vi "Check and send command to corresponding device.vi"(8 "error in (no error)":errorcluster, 9 "Execute cmd (F)":bool, 10 "Cmd string":string="power -10 0") -> (0 "error out":errorcluster, 3 "Response":string)   [LabVIEW 2019]
doc: "Nicolas Weiss - EPFL - IPHYS 2019\n----\nThis VI :\n- parses a user command\n- checks syntax and arguments validity\n- sends it to the corresponding device"
uses:
  Controls/Log destination selector.ctl
  Controls/Lakeshore device selector.ctl
  _Global variables 1.vi
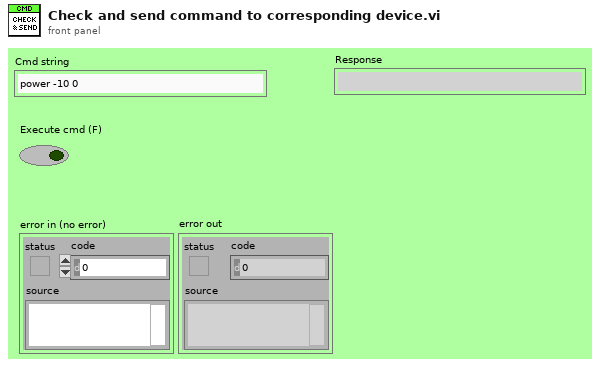
[diagram p1: front panel]
types:
  T1 = typedef "Log destination selector.ctl" = enum16{"UI", "File", "UI+file"}
  T2 = typedef "Lakeshore device selector.ctl" = enum16{"A", "B"}
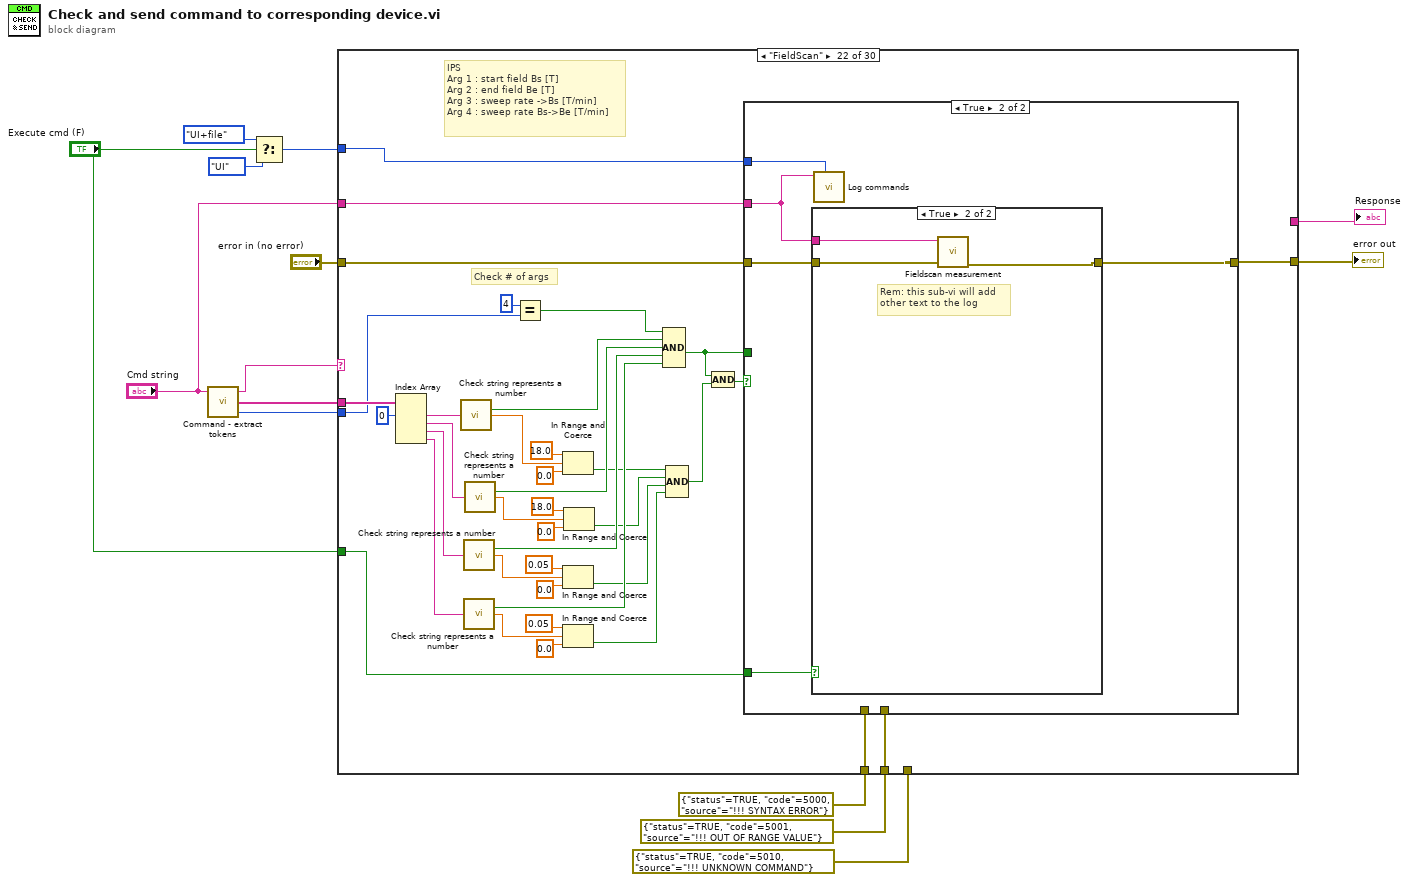
[diagram p0: block diagram]
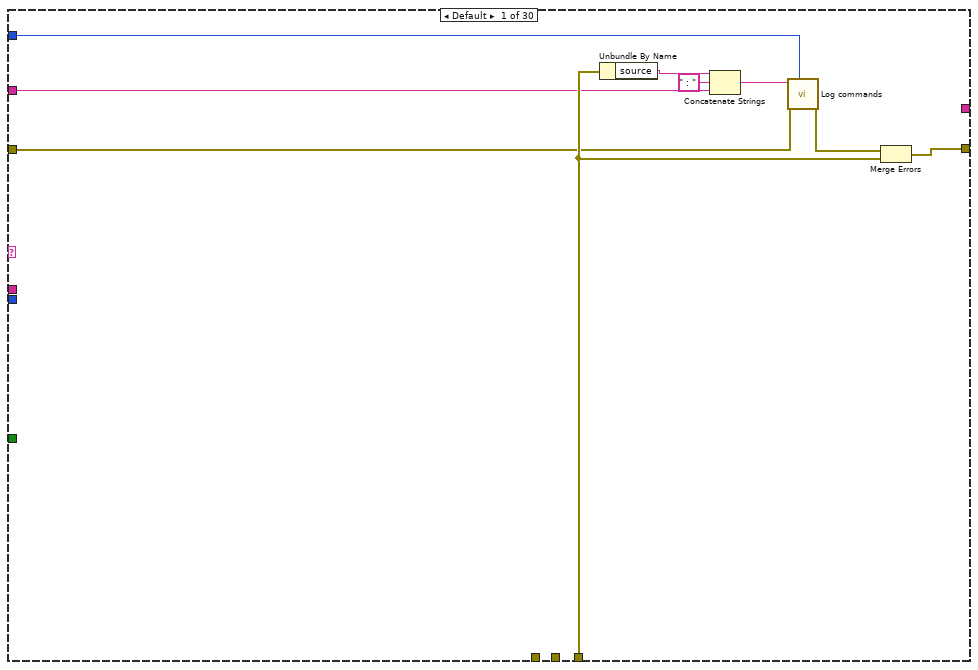
[diagram p2: hidden frame]
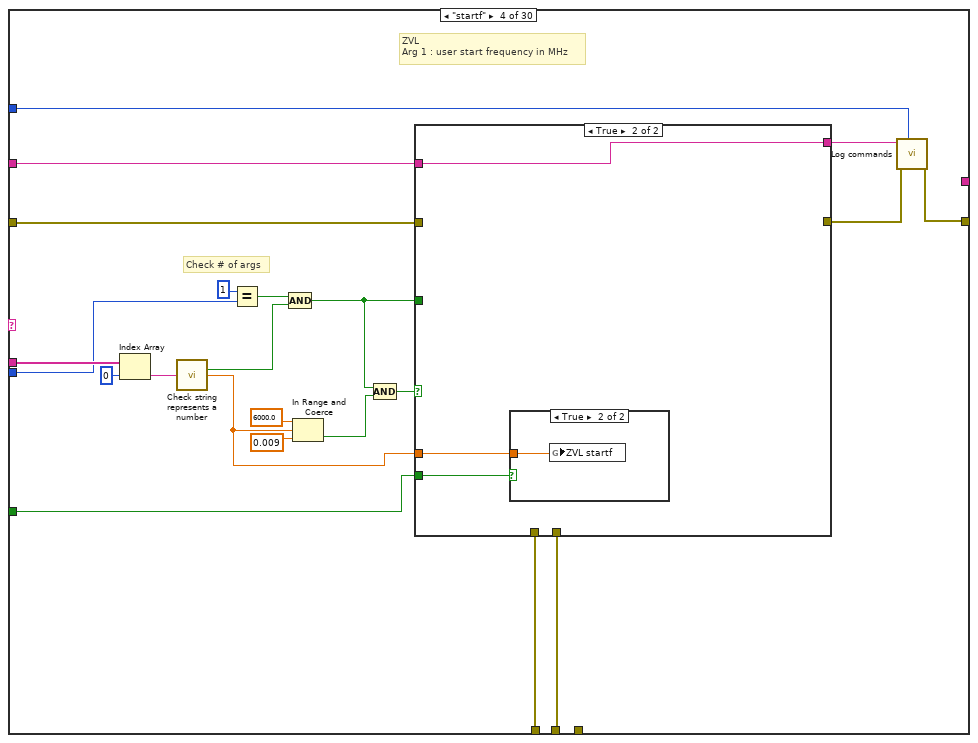
[diagram p5: hidden frame]
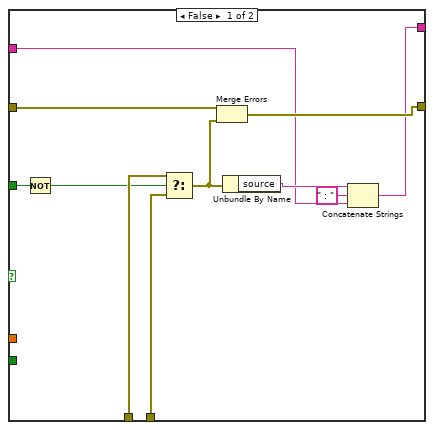
[diagram p6: hidden frame]
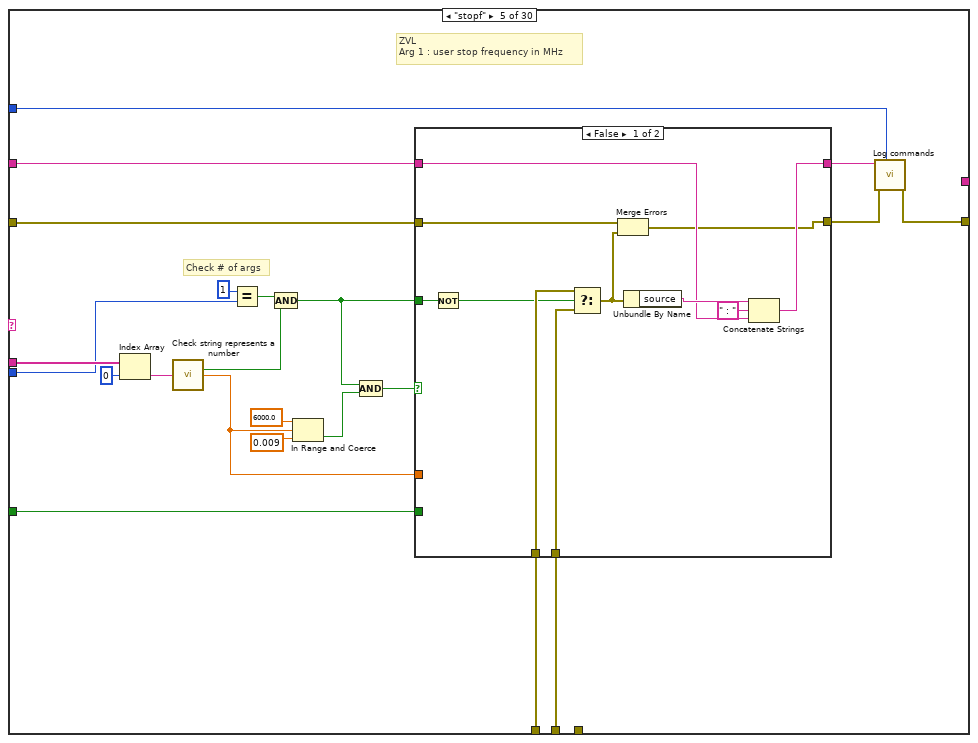
[diagram p8: hidden frame]
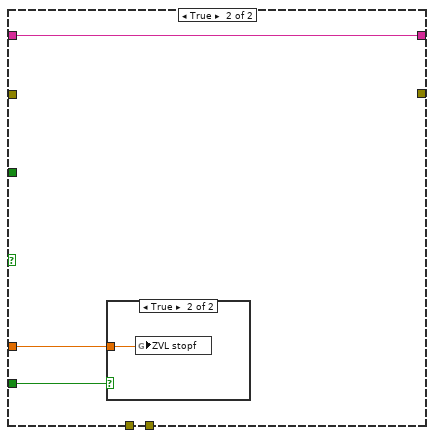
[diagram p9: hidden frame]
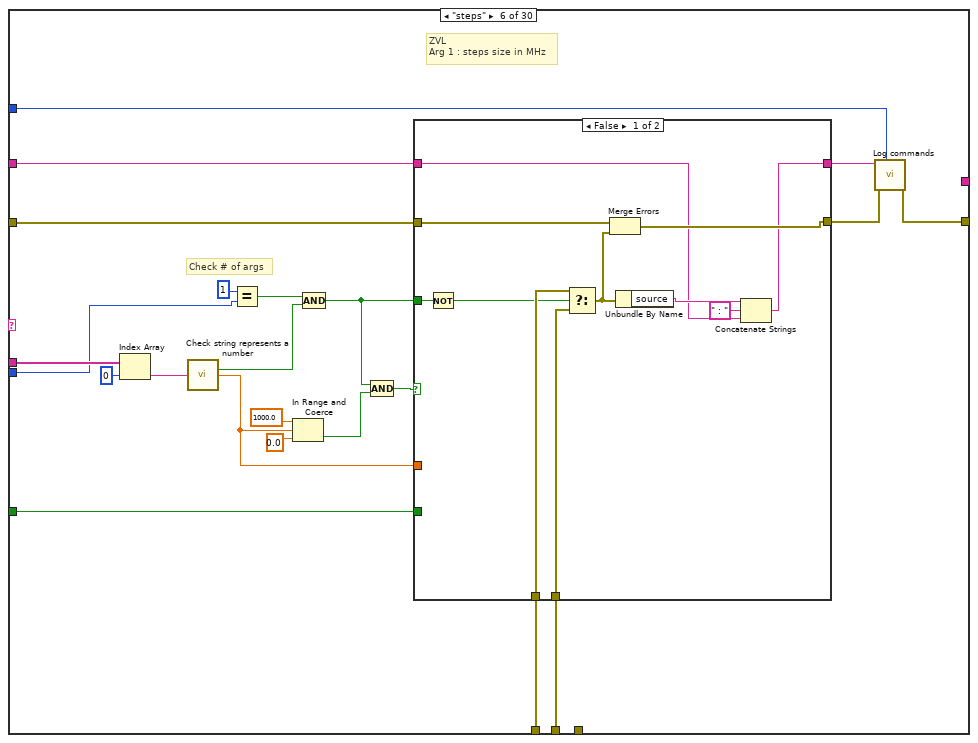
[diagram p11: hidden frame]
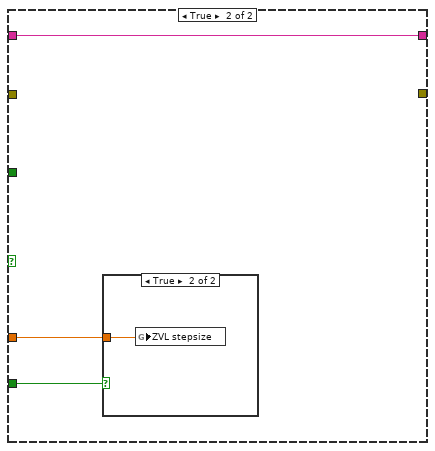
[diagram p12: hidden frame]
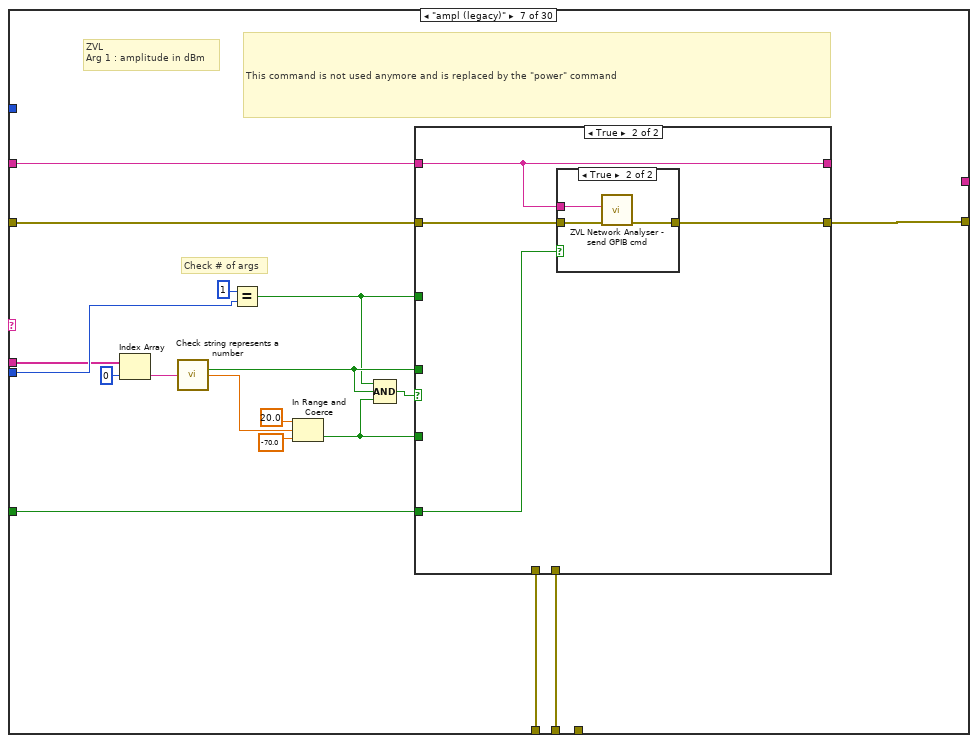
[diagram p14: hidden frame]
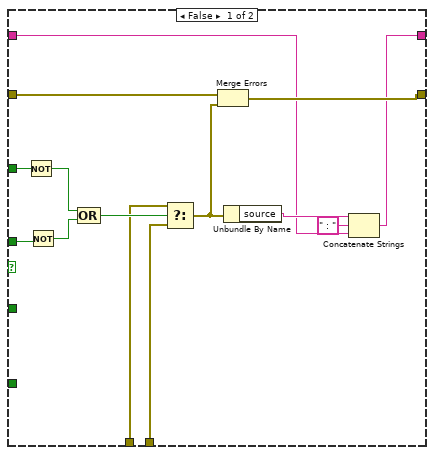
[diagram p15: hidden frame]
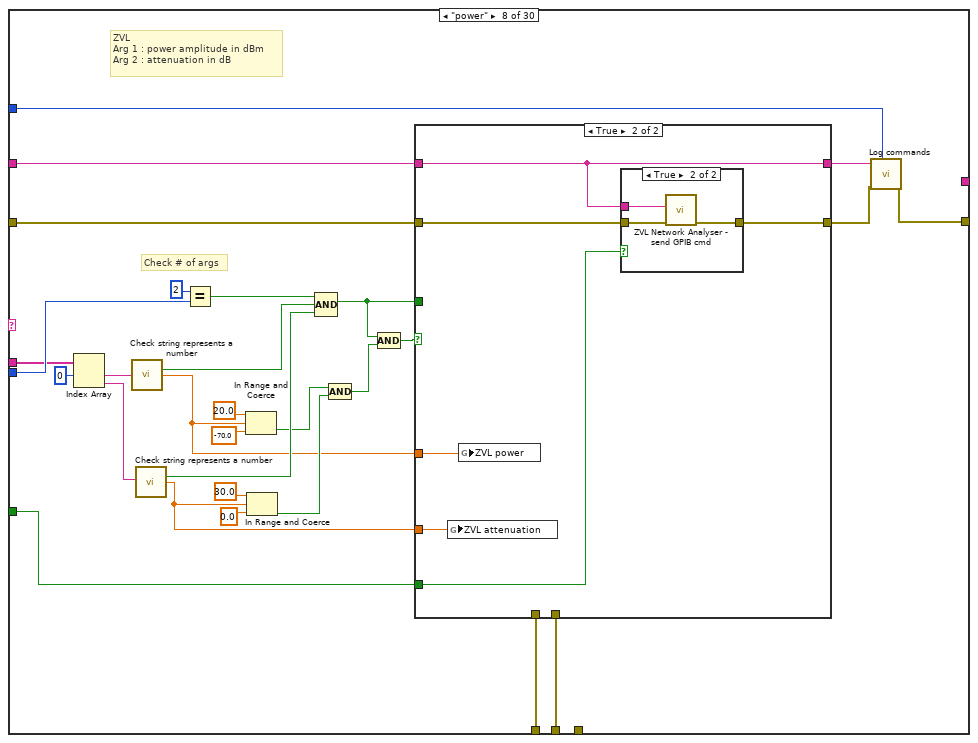
[diagram p17: hidden frame]
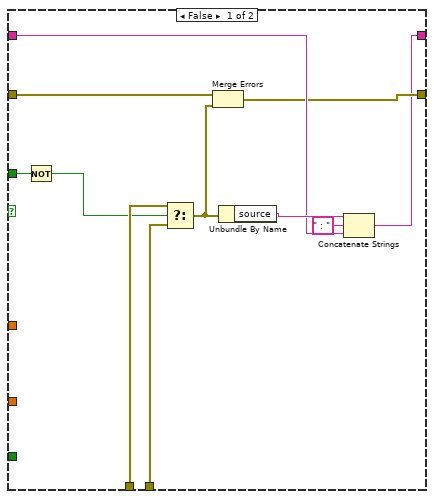
[diagram p18: hidden frame]
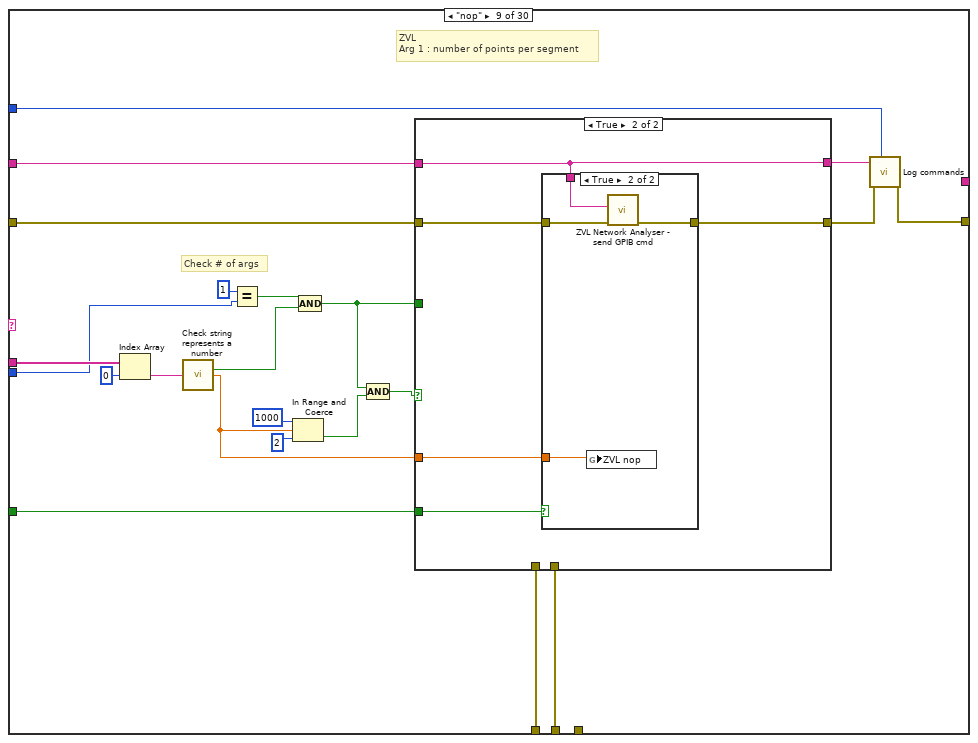
[diagram p20: hidden frame]
diagram:
  n1 = call "Command - extract tokens.vi"("Cmd string"="Cmd string") -> ("N arg"=w8:u8, "Arguments"=w11:string[], "Command"=w9:string)  [unwired: 2 in]
  n2 = Select(t=Log_destination_selector."UI+file" ("Log destination"), s="Execute cmd (F)", f=Log_destination_selector."UI" ("Log destination")) -> (s? t:f=w1:T1)
  n3 = case shown="\"FieldScan\"" w9 {
    tunnel: w11 -> [_ _ _ w46 w83 w120 w151 w199 w247 _ _ _ w308 w348 w383 _ _ _ _ _ _ w596 _ w647 w687 _ _ _ _ _]
    tunnel: w8 -> [_ _ _ w44 w82 w119 w154 w204 w246 _ _ _ w307 w347 w382 w411 w438 w467 w496 w524 w550 w585 _ w646 w686 _ _ _ _ _]
    tunnel: "error in (no error)" -> [w16 w24 w25 w40 w78 w115 w153 w200 w242 w272 w281 w287 w303 w343 w380 w409 w436 w465 w494 w522 w548 w598 w626 w642 w682 w710 w720 w727 w728 w729]
    tunnel: [w23 w24 w25 w30 w68 w105 w152 w177 w232 w271 w280 w287 w293 w333 w372 w401 w428 w457 w486 w514 w540 w597 w626 w632 w672 w709 w719 w727 w728 w729] -> w13
    tunnel: [_ _ _ _ _ _ _ _ _ w270 w279 _ _ _ _ _ w426 w455 w484 _ _ _ _ _ _ w708 w718 _ _ _] -> w12
    tunnel: "Cmd string" -> [w19 _ _ w39 w77 w114 w150 w198 w241 _ _ _ w302 w342 w379 w408 w435 w464 w493 w521 w547 w595 _ w641 w681 _ _ _ _ _]
    tunnel: "Execute cmd (F)" -> [_ _ _ w38 w76 w113 w149 w197 w240 w269 w278 _ w301 w341 w378 w407 w434 w463 w492 w520 w546 w594 _ w640 w680 w707 w717 _ _ _]
    tunnel: errorcluster {"status"=TRUE, "code"=5001, "source"="!!! OUT OF RANGE VALUE"} ("error out") -> [_ _ _ w34 w72 w110 w147 w194 w236 _ _ _ w297 w337 w376 w405 w432 w461 w490 w518 w544 w590 _ w636 w676 _ _ _ _ _]
    tunnel: errorcluster {"status"=TRUE, "code"=5000, "source"="!!! SYNTAX ERROR"} ("error out") -> [_ _ _ w35 w73 w109 w148 w195 w237 _ _ _ w298 w338 w377 w406 w433 w462 w491 w519 w545 w591 _ w637 w677 _ _ _ _ _]
    tunnel: errorcluster {"status"=TRUE, "code"=5010, "source"="!!! UNKNOWN COMMAND"} ("error out") -> [w20 _ _ _ _ _ _ _ _ _ _ _ _ _ _ _ _ _ _ _ _ _ _ _ _ _ _ _ _ _]
    tunnel: w1 -> [w17 _ _ w32 w70 w107 _ w179 w234 _ _ _ w295 w335 w374 w403 w430 w459 w488 w516 w542 w565 _ w634 w674 _ _ _ _ _]
    frame Default {
      n4 = Unbundle By Name(w20) -> ("source"=w22:string)
      n5 = Concatenate Strings(w22, " : " ("string"), w19) -> (w18:string)
      n6 = call "Log commands.vi"("Log destination"=w17, "error in"=w16, "text to log"=w18) -> ("error out"=w15:errorcluster)  [unwired: 8 in]
      n7 = Merge Errors(w15, w20) -> (w23:errorcluster)
    }
    frame "#", "%", "//", "rem" {
      # "Commented line"
    }
    frame "--- ZVL ---" {
      # "separator"
    }
    frame "startf" {
      # "Check # of args"
      # "ZVL\nArg 1 : user start frequency in MHz"
      n8 = Index Array(array=w46, index=0) -> (element=w37:string)
      n9 = call "Check string represents a number.vi"("String"=w37) -> ("Is a number"=w28:bool, "Number"=w36:dbl)  [unwired: 13 in]
      n10 = Equal?(x=1 ("y"), y=w44) -> (x = y?=w29:bool)
      n11 = Compound Arithmetic op=AND(w29, w28) -> (w26:bool)
      n12 = In Range and Coerce(upper limit=6000.0 ("lower limit"), x=w36, lower limit=0.009) -> (In Range?=w27:bool)  [unwired: 1 out]
      n13 = Compound Arithmetic op=AND(w26, w27) -> (w45:bool)
      n14 = case shown="True" w45 {
        tunnel: w36 -> [_ w61]
        tunnel: w40 -> [w58 _]
        tunnel: [w57 _] -> w31
        tunnel: w39 -> [w50 w60]
        tunnel: [w49 w60] -> w33
        tunnel: w38 -> [_ w59]
        tunnel: w26 -> [w56 _]
        tunnel: w35 -> [w55 _]
        tunnel: w34 -> [w54 _]
        frame False {
          n15 = Not(x=w56) -> (.not. x?=w48:bool)
          n16 = Select(t=w55, s=w48, f=w54) -> (s? t:f=w51:errorcluster)
          n17 = Merge Errors(w58, w51) -> (w57:errorcluster)
          n18 = Unbundle By Name(w51) -> ("source"=w52:string)
          n19 = Concatenate Strings(w52, " : " ("string"), w50) -> (w49:string)
        }
        frame True {
          n20 = case shown="True" w59 {
            tunnel: w61 -> [_ w62]
            frame False {
            }
            frame True {
              n21 = global write "_Global variables 1.vi" "ZVL startf"(w62) -> ()
            }
          }
        }
      }
      n22 = call "Log commands.vi"("Log destination"=w32, "error in"=w31, "text to log"=w33) -> ("error out"=w30:errorcluster)  [unwired: 8 in]
    }
    frame "stopf" {
      # "Check # of args"
      # "ZVL\nArg 1 : user stop frequency in MHz"
      n23 = Index Array(array=w83, index=0) -> (element=w75:string)
      n24 = call "Check string represents a number.vi"("String"=w75) -> ("Is a number"=w66:bool, "Number"=w74:dbl)  [unwired: 13 in]
      n25 = Equal?(x=1 ("y"), y=w82) -> (x = y?=w67:bool)
      n26 = Compound Arithmetic op=AND(w67, w66) -> (w65:bool)
      n27 = In Range and Coerce(upper limit=6000.0 ("lower limit"), x=w74, lower limit=0.009) -> (In Range?=w64:bool)  [unwired: 1 out]
      n28 = Compound Arithmetic op=AND(w65, w64) -> (w63:bool)
      n29 = case shown="False" w63 {
        tunnel: [w89 w97] -> w71
        tunnel: w74 -> [_ w98]
        tunnel: w78 -> [w87 _]
        tunnel: [w88 _] -> w69
        tunnel: w77 -> [w90 w97]
        tunnel: w76 -> [_ w96]
        tunnel: w65 -> [w95 _]
        tunnel: w73 -> [w94 _]
        tunnel: w72 -> [w93 _]
        frame False {
          n30 = Not(x=w95) -> (.not. x?=w85:bool)
          n31 = Select(t=w94, s=w85, f=w93) -> (s? t:f=w86:errorcluster)
          n32 = Merge Errors(w87, w86) -> (w88:errorcluster)
          n33 = Unbundle By Name(w86) -> ("source"=w91:string)
          n34 = Concatenate Strings(w91, " : " ("string"), w90) -> (w89:string)
        }
        frame True {
          n35 = case shown="True" w96 {
            tunnel: w98 -> [_ w99]
            frame False {
            }
            frame True {
              n36 = global write "_Global variables 1.vi" "ZVL stopf"(w99) -> ()
            }
          }
        }
      }
      n37 = call "Log commands.vi"("Log destination"=w70, "error in"=w69, "text to log"=w71) -> ("error out"=w68:errorcluster)  [unwired: 8 in]
    }
    frame "steps" {
      # "Check # of args"
      # "ZVL\nArg 1 : steps size in MHz"
      n38 = Index Array(array=w120, index=0) -> (element=w112:string)
      n39 = call "Check string represents a number.vi"("String"=w112) -> ("Is a number"=w103:bool, "Number"=w111:dbl)  [unwired: 13 in]
      n40 = Equal?(x=1 ("y"), y=w119) -> (x = y?=w104:bool)
      n41 = In Range and Coerce(upper limit=1000.0 ("lower limit"), x=w111, lower limit=0.0) -> (In Range?=w100:bool)  [unwired: 1 out]
      n42 = Compound Arithmetic op=AND(w104, w103) -> (w102:bool)
      n43 = Compound Arithmetic op=AND(w102, w100) -> (w101:bool)
      n44 = case shown="False" w101 {
        tunnel: w111 -> [_ w135]
        tunnel: w115 -> [w126 _]
        tunnel: [w125 _] -> w106
        tunnel: w114 -> [w123 w134]
        tunnel: [w124 w134] -> w108
        tunnel: w113 -> [_ w133]
        tunnel: w102 -> [w132 _]
        tunnel: w110 -> [w131 _]
        tunnel: w109 -> [w130 _]
        frame False {
          n45 = Not(x=w132) -> (.not. x?=w122:bool)
          n46 = Select(t=w130, s=w122, f=w131) -> (s? t:f=w127:errorcluster)
          n47 = Merge Errors(w126, w127) -> (w125:errorcluster)
          n48 = Unbundle By Name(w127) -> ("source"=w128:string)
          n49 = Concatenate Strings(w128, " : " ("string"), w123) -> (w124:string)
        }
        frame True {
          n50 = case shown="True" w133 {
            tunnel: w135 -> [_ w136]
            frame False {
            }
            frame True {
              n51 = global write "_Global variables 1.vi" "ZVL stepsize"(w136) -> ()
            }
          }
        }
      }
      n52 = call "Log commands.vi"("Log destination"=w107, "error in"=w106, "text to log"=w108) -> ("error out"=w105:errorcluster)  [unwired: 8 in]
    }
    frame "ampl (legacy)" {
      # "Check # of args"
      # "This command is not used anymore and is replaced by the \"power\" command"
      # "ZVL\nArg 1 : amplitude in dBm"
      n53 = Index Array(array=w151, index=0) -> (element=w140:string)
      n54 = call "Check string represents a number.vi"("String"=w140) -> ("Is a number"=w139:bool, "Number"=w138:dbl)  [unwired: 13 in]
      n55 = Equal?(x=1 ("y"), y=w154) -> (x = y?=w137:bool)
      n56 = In Range and Coerce(upper limit=20.0 ("lower limit"), x=w138, lower limit=-70.0) -> (In Range?=w141:bool)  [unwired: 1 out]
      n57 = Compound Arithmetic op=AND(w137, w139, w141) -> (w145:bool)
      n58 = case shown="True" w145 {
        tunnel: w141 -> [_ _]
        tunnel: w153 -> [w158 w171]
        tunnel: [w157 w172] -> w152
        tunnel: [w156 w170] -> _
        tunnel: w150 -> [w155 w170]
        tunnel: w149 -> [_ w169]
        tunnel: w139 -> [w164 _]
        tunnel: w137 -> [w165 _]
        tunnel: w148 -> [w163 _]
        tunnel: w147 -> [w162 _]
        frame False {
          n59 = Not(x=w165) -> (.not. x?=w167:bool)
          n60 = Not(x=w164) -> (.not. x?=w166:bool)
          n61 = Compound Arithmetic op=OR(w167, w166) -> (w168:bool)
          n62 = Select(t=w163, s=w168, f=w162) -> (s? t:f=w159:errorcluster)
          n63 = Merge Errors(w158, w159) -> (w157:errorcluster)
          n64 = Unbundle By Name(w159) -> ("source"=w160:string)
          n65 = Concatenate Strings(w160, " : " ("string"), w155) -> (w156:string)
        }
        frame True {
          n66 = case shown="True" w169 {
            tunnel: [w173 w176] -> w172
            tunnel: w171 -> [w173 w175]
            tunnel: w170 -> [_ w174]
            frame False {
            }
            frame True {
              n67 = call "ZVL Network Analyser - send GPIB cmd.vi"("error in (no error)"=w175, "Cmd string"=w174) -> ("error out"=w176:errorcluster)  [unwired: 8 in, 1 out]
            }
          }
        }
      }
    }
    frame "power" {
      # "Check # of args"
      # "ZVL\nArg 1 : power amplitude in dBm\nArg 2 : attenuation in dB"
      n68 = Index Array(array=w199, index #1=0 ("index")) -> (element #1=w196:string, element #2=w193:string)  [unwired: 1 in]
      n69 = call "Check string represents a number.vi"("String"=w196) -> ("Is a number"=w188:bool, "Number"=w182:dbl)  [unwired: 13 in]
      n70 = call "Check string represents a number.vi"("String"=w193) -> ("Is a number"=w187:bool, "Number"=w181:dbl)  [unwired: 13 in]
      n71 = Equal?(x=2 ("y"), y=w204) -> (x = y?=w189:bool)
      n72 = In Range and Coerce(upper limit=20.0 ("lower limit"), x=w182, lower limit=-70.0) -> (In Range?=w186:bool)  [unwired: 1 out]
      n73 = In Range and Coerce(upper limit=30.0 ("lower limit"), x=w181, lower limit=0.0) -> (In Range?=w185:bool)  [unwired: 1 out]
      n74 = Compound Arithmetic op=AND(w189, w188, w187) -> (w183:bool)
      n75 = Compound Arithmetic op=AND(w186, w185) -> (w190:bool)
      n76 = Compound Arithmetic op=AND(w183, w190) -> (w184:bool)
      n77 = case shown="True" w184 {
        tunnel: w200 -> [w210 w221]
        tunnel: [w208 w222] -> w178
        tunnel: [w207 w220] -> w180
        tunnel: w198 -> [w209 w220]
        tunnel: w197 -> [_ w219]
        tunnel: w183 -> [w216 _]
        tunnel: w195 -> [w215 _]
        tunnel: w194 -> [w214 _]
        tunnel: w182 -> [_ w218]
        tunnel: w181 -> [_ w217]
        frame False {
          n78 = Not(x=w216) -> (.not. x?=w206:bool)
          n79 = Select(t=w215, s=w206, f=w214) -> (s? t:f=w211:errorcluster)
          n80 = Merge Errors(w210, w211) -> (w208:errorcluster)
          n81 = Unbundle By Name(w211) -> ("source"=w212:string)
          n82 = Concatenate Strings(w212, " : " ("string"), w209) -> (w207:string)
        }
        frame True {
          n83 = global write "_Global variables 1.vi" "ZVL attenuation"(w217) -> ()
          n84 = global write "_Global variables 1.vi" "ZVL power"(w218) -> ()
          n85 = case shown="True" w219 {
            tunnel: [w223 w226] -> w222
            tunnel: w221 -> [w223 w225]
            tunnel: w220 -> [_ w224]
            frame False {
            }
            frame True {
              n86 = call "ZVL Network Analyser - send GPIB cmd.vi"("error in (no error)"=w225, "Cmd string"=w224) -> ("error out"=w226:errorcluster)  [unwired: 8 in, 1 out]
            }
          }
        }
      }
      n87 = call "Log commands.vi"("Log destination"=w179, "error in"=w178, "text to log"=w180) -> ("error out"=w177:errorcluster)  [unwired: 8 in]
    }
    frame "nop" {
      # "Check # of args"
      # "ZVL\nArg 1 : number of points per segment"
      n88 = Index Array(array=w247, index=0) -> (element=w239:string)
      n89 = call "Check string represents a number.vi"("String"=w239) -> ("Is a number"=w230:bool, "Number"=w238:dbl)  [unwired: 13 in]
      n90 = Equal?(x=1 ("y"), y=w246) -> (x = y?=w231:bool)
      n91 = In Range and Coerce(upper limit=1000 ("lower limit"), x=w238, lower limit=2) -> (In Range?=w227:bool)  [unwired: 1 out]
      n92 = Compound Arithmetic op=AND(w231, w230) -> (w229:bool)
      n93 = Compound Arithmetic op=AND(w229, w227) -> (w228:bool)
      n94 = case shown="True" w228 {
        tunnel: [w251 w261] -> w235
        tunnel: w238 -> [_ w260]
        tunnel: w242 -> [w253 w263]
        tunnel: [w253 w262] -> w233
        tunnel: w241 -> [w252 w261]
        tunnel: w240 -> [_ w259]
        tunnel: w237 -> [w258 _]
        tunnel: w236 -> [w257 _]
        tunnel: w229 -> [w250 _]
        frame False {
          n95 = Not(x=w250) -> (.not. x?=w249:bool)
          n96 = Select(t=w258, s=w249, f=w257) -> (s? t:f=w254:errorcluster)
          n97 = Merge Errors(w253, w254) -> ()  [unwired: 1 out]
          n98 = Unbundle By Name(w254) -> ("source"=w255:string)
          n99 = Concatenate Strings(w255, " : " ("string"), w252) -> (w251:string)
        }
        frame True {
          n100 = case shown="True" w259 {
            tunnel: w263 -> [w264 w268]
            tunnel: [w264 w267] -> w262
            tunnel: w261 -> [_ w266]
            tunnel: w260 -> [_ w265]
            frame False {
            }
            frame True {
              n101 = global write "_Global variables 1.vi" "ZVL nop"(w265) -> ()
              n102 = call "ZVL Network Analyser - send GPIB cmd.vi"("error in (no error)"=w268, "Cmd string"=w266) -> ("error out"=w267:errorcluster)  [unwired: 8 in, 1 out]
            }
          }
        }
      }
      n103 = call "Log commands.vi"("Log destination"=w234, "error in"=w233, "text to log"=w235) -> ("error out"=w232:errorcluster)  [unwired: 8 in]
    }
    frame "Get_ZVL_ACfield" {
      # "ZVL\nInput : no argument"
      n104 = case shown="True" w269 {
        tunnel: w272 -> [w273 w277]
        tunnel: [w273 w276] -> w271
        tunnel: [_ w275] -> w270
        frame False {
        }
        frame True {
          n105 = call "ZVL Network Analyser - send GPIB cmd.vi"("error in (no error)"=w277, "Cmd string"="readSdat1") -> ("error out"=w276:errorcluster, "Response"=w275:string)  [unwired: 8 in]
        }
      }
    }
    frame "Get_ZVL_data" {
      # "ZVL\nInput : no argument"
      n106 = case shown="True" w278 {
        tunnel: w281 -> [w282 w286]
        tunnel: [w282 w285] -> w280
        tunnel: [_ w284] -> w279
        frame False {
        }
        frame True {
          n107 = call "ZVL Network Analyser - send GPIB cmd.vi"("error in (no error)"=w286, "Cmd string"="readStim1") -> ("error out"=w285:errorcluster, "Response"=w284:string)  [unwired: 8 in]
        }
      }
    }
    frame "--- IPS ---" {
      # "separator"
    }
    frame "FieldRate" {
      # "Check # of args"
      # "IPS\nArg 1 : field sweep rate [T/min]"
      n108 = Index Array(array=w308, index=0) -> (element=w300:string)
      n109 = call "Check string represents a number.vi"("String"=w300) -> ("Is a number"=w291:bool, "Number"=w299:dbl)  [unwired: 13 in]
      n110 = Equal?(x=1 ("y"), y=w307) -> (x = y?=w292:bool)
      n111 = In Range and Coerce(upper limit=0.1 ("lower limit"), x=w299, lower limit=0.001) -> (In Range?=w288:bool)  [unwired: 1 out]
      n112 = Compound Arithmetic op=AND(w292, w291) -> (w290:bool)
      n113 = Compound Arithmetic op=AND(w290, w288) -> (w289:bool)
      n114 = case shown="True" w289 {
        tunnel: [w312 w321] -> w296
        tunnel: w303 -> [w314 w323]
        tunnel: [w314 w322] -> w294
        tunnel: w302 -> [w313 w321]
        tunnel: w301 -> [_ w320]
        tunnel: w298 -> [w319 _]
        tunnel: w297 -> [w318 _]
        tunnel: w290 -> [w311 _]
        frame False {
          n115 = Not(x=w311) -> (.not. x?=w310:bool)
          n116 = Select(t=w319, s=w310, f=w318) -> (s? t:f=w315:errorcluster)
          n117 = Merge Errors(w314, w315) -> ()  [unwired: 1 out]
          n118 = Unbundle By Name(w315) -> ("source"=w316:string)
          n119 = Concatenate Strings(w316, " : " ("string"), w313) -> (w312:string)
        }
        frame True {
          n120 = case shown="True" w320 {
            tunnel: w323 -> [w324 w327]
            tunnel: [w324 w326] -> w322
            tunnel: w321 -> [_ w325]
            frame False {
            }
            frame True {
              n121 = call "IPS magnet power supply - send GPIB cmd.vi"("error in (no error)"=w327, "Cmd string"=w325) -> ("error out"=w326:errorcluster)  [unwired: 8 in, 1 out]
            }
          }
        }
      }
      n122 = call "Log commands.vi"("Log destination"=w295, "error in"=w294, "text to log"=w296) -> ("error out"=w293:errorcluster)  [unwired: 8 in]
    }
    frame "FieldSetpoint" {
      # "Check # of args"
      # "IPS\nArg 1 : magnetic field target in T"
      n123 = Index Array(array=w348, index=0) -> (element=w340:string)
      n124 = call "Check string represents a number.vi"("String"=w340) -> ("Is a number"=w331:bool, "Number"=w339:dbl)  [unwired: 13 in]
      n125 = Equal?(x=1 ("y"), y=w347) -> (x = y?=w332:bool)
      n126 = In Range and Coerce(upper limit=18.0 ("lower limit"), x=w339, lower limit=0.0) -> (In Range?=w328:bool)  [unwired: 1 out]
      n127 = Compound Arithmetic op=AND(w332, w331) -> (w330:bool)
      n128 = Compound Arithmetic op=AND(w330, w328) -> (w329:bool)
      n129 = case shown="True" w329 {
        tunnel: [w352 w361] -> w336
        tunnel: w343 -> [w354 w363]
        tunnel: [w354 w362] -> w334
        tunnel: w342 -> [w353 w361]
        tunnel: w341 -> [_ w360]
        tunnel: w338 -> [w359 _]
        tunnel: w337 -> [w358 _]
        tunnel: w330 -> [w351 _]
        frame False {
          n130 = Not(x=w351) -> (.not. x?=w350:bool)
          n131 = Select(t=w359, s=w350, f=w358) -> (s? t:f=w355:errorcluster)
          n132 = Merge Errors(w354, w355) -> ()  [unwired: 1 out]
          n133 = Unbundle By Name(w355) -> ("source"=w356:string)
          n134 = Concatenate Strings(w356, " : " ("string"), w353) -> (w352:string)
        }
        frame True {
          n135 = case shown="True" w360 {
            tunnel: w363 -> [w364 w367]
            tunnel: [w364 w366] -> w362
            tunnel: w361 -> [_ w365]
            frame False {
            }
            frame True {
              n136 = call "IPS magnet power supply - send GPIB cmd.vi"("error in (no error)"=w367, "Cmd string"=w365) -> ("error out"=w366:errorcluster)  [unwired: 8 in, 1 out]
            }
          }
        }
      }
      n137 = call "Log commands.vi"("Log destination"=w335, "error in"=w334, "text to log"=w336) -> ("error out"=w333:errorcluster)  [unwired: 8 in]
    }
    frame "IPSheater" {
      # "Check # of args"
      # "IPS\nArg 1 : on|off heater state"
      n138 = Index Array(array=w383, index=0) -> (element=w370:string)
      n139 = case shown="Default" w370 {
        tunnel: [_ TRUE ("status")] -> w369
        frame Default {
        }
        frame "off", "on" {
        }
      }
      n140 = Equal?(x=1 ("y"), y=w382) -> (x = y?=w371:bool)
      n141 = Compound Arithmetic op=AND(w371, w369) -> (w368:bool)
      n142 = case shown="True" w368 {
        tunnel: [w387 w393] -> w375
        tunnel: w380 -> [w389 w395]
        tunnel: [w389 w394] -> w373
        tunnel: w379 -> [w388 w393]
        tunnel: w378 -> [_ w392]
        tunnel: w377 -> [w386 _]
        tunnel: w376 -> [_ _]
        frame False {
          n143 = Merge Errors(w389, w386) -> ()  [unwired: 1 out]
          n144 = Unbundle By Name(w386) -> ("source"=w390:string)
          n145 = Concatenate Strings(w390, " : " ("string"), w388) -> (w387:string)
        }
        frame True {
          n146 = case shown="True" w392 {
            tunnel: w395 -> [w396 w399]
            tunnel: [w396 w398] -> w394
            tunnel: w393 -> [_ w397]
            frame False {
            }
            frame True {
              n147 = call "IPS magnet power supply - send GPIB cmd.vi"("error in (no error)"=w399, "Cmd string"=w397) -> ("error out"=w398:errorcluster)  [unwired: 8 in, 1 out]
            }
          }
        }
      }
      n148 = call "Log commands.vi"("Log destination"=w374, "error in"=w373, "text to log"=w375) -> ("error out"=w372:errorcluster)  [unwired: 8 in]
    }
    frame "GetFieldSetpoint" {
      # "Check # of args"
      # "IPS\nNo arg\nResponse : setpoint field in T"
      n149 = Equal?(x=0 ("y"), y=w411) -> (x = y?=w400:bool)
      n150 = case shown="True" w400 {
        tunnel: [w413 w419] -> w404
        tunnel: w409 -> [w415 w421]
        tunnel: [w415 w420] -> w402
        tunnel: w408 -> [w414 w419]
        tunnel: w407 -> [_ w418]
        tunnel: w406 -> [w412 _]
        tunnel: w405 -> [_ _]
        frame False {
          n151 = Merge Errors(w415, w412) -> ()  [unwired: 1 out]
          n152 = Unbundle By Name(w412) -> ("source"=w416:string)
          n153 = Concatenate Strings(w416, " : " ("string"), w414) -> (w413:string)
        }
        frame True {
          n154 = case shown="True" w418 {
            tunnel: w421 -> [w422 w425]
            tunnel: [w422 w424] -> w420
            tunnel: w419 -> [_ w423]
            frame False {
            }
            frame True {
              n155 = call "IPS magnet power supply - send GPIB cmd.vi"("error in (no error)"=w425, "Cmd string"=w423) -> ("error out"=w424:errorcluster)  [unwired: 8 in, 1 out]
            }
          }
        }
      }
      n156 = call "Log commands.vi"("Log destination"=w403, "error in"=w402, "text to log"=w404) -> ("error out"=w401:errorcluster)  [unwired: 8 in]
    }
    frame "ToFieldSetpoint" {
      # "IPS\nNo arg\nResponse : field setpoint"
      # "Check # of args"
      n157 = Equal?(x=0 ("y"), y=w438) -> (x = y?=w427:bool)
      n158 = case shown="True" w427 {
        tunnel: [w440 w447] -> w431
        tunnel: w436 -> [w442 w449]
        tunnel: [w442 w448] -> w429
        tunnel: w435 -> [w441 w447]
        tunnel: w434 -> [_ w446]
        tunnel: w433 -> [w439 _]
        tunnel: w432 -> [_ _]
        tunnel: [_ w445] -> w426
        frame False {
          n159 = Merge Errors(w442, w439) -> ()  [unwired: 1 out]
          n160 = Unbundle By Name(w439) -> ("source"=w443:string)
          n161 = Concatenate Strings(w443, " : " ("string"), w441) -> (w440:string)
        }
        frame True {
          n162 = case shown="True" w446 {
            tunnel: w449 -> [w450 w454]
            tunnel: [w450 w453] -> w448
            tunnel: w447 -> [_ w452]
            tunnel: [_ w451] -> w445
            frame False {
            }
            frame True {
              n163 = call "IPS magnet power supply - send GPIB cmd.vi"("error in (no error)"=w454, "Cmd string"=w452) -> ("error out"=w453:errorcluster, "Response"=w451:string)  [unwired: 8 in]
            }
          }
        }
      }
      n164 = call "Log commands.vi"("Log destination"=w430, "error in"=w429, "text to log"=w431) -> ("error out"=w428:errorcluster)  [unwired: 8 in]
    }
    frame "GetField" {
      # "IPS\nNo arg\nResponse : magnetic field in T"
      # "Check # of args"
      n165 = Equal?(x=0 ("y"), y=w467) -> (x = y?=w456:bool)
      n166 = case shown="True" w456 {
        tunnel: [w469 w476] -> w460
        tunnel: w465 -> [w471 w478]
        tunnel: [w471 w477] -> w458
        tunnel: w464 -> [w470 w476]
        tunnel: w463 -> [_ w475]
        tunnel: w462 -> [w468 _]
        tunnel: w461 -> [_ _]
        tunnel: [_ w474] -> w455
        frame False {
          n167 = Merge Errors(w471, w468) -> ()  [unwired: 1 out]
          n168 = Unbundle By Name(w468) -> ("source"=w472:string)
          n169 = Concatenate Strings(w472, " : " ("string"), w470) -> (w469:string)
        }
        frame True {
          n170 = case shown="True" w475 {
            tunnel: w478 -> [w479 w483]
            tunnel: [w479 w482] -> w477
            tunnel: w476 -> [_ w481]
            tunnel: [_ w480] -> w474
            frame False {
            }
            frame True {
              n171 = call "IPS magnet power supply - send GPIB cmd.vi"("error in (no error)"=w483, "Cmd string"=w481) -> ("error out"=w482:errorcluster, "Response"=w480:string)  [unwired: 8 in]
            }
          }
        }
      }
      n172 = call "Log commands.vi"("Log destination"=w459, "error in"=w458, "text to log"=w460) -> ("error out"=w457:errorcluster)  [unwired: 8 in]
    }
    frame "IPSstatus" {
      # "IPS\nNo arg\nResponse : status code (Xmn An Cn Hn Mmn Pmn)\nRem : the responded status is also written in the global varaible cluster"
      # "Check # of args"
      n173 = Equal?(x=0 ("y"), y=w496) -> (x = y?=w485:bool)
      n174 = case shown="True" w485 {
        tunnel: [w498 w505] -> w489
        tunnel: w494 -> [w500 w507]
        tunnel: [w500 w506] -> w487
        tunnel: w493 -> [w499 w505]
        tunnel: w492 -> [_ w504]
        tunnel: w491 -> [w497 _]
        tunnel: w490 -> [_ _]
        tunnel: [_ w503] -> w484
        frame False {
          n175 = Merge Errors(w500, w497) -> ()  [unwired: 1 out]
          n176 = Unbundle By Name(w497) -> ("source"=w501:string)
          n177 = Concatenate Strings(w501, " : " ("string"), w499) -> (w498:string)
        }
        frame True {
          n178 = case shown="True" w504 {
            tunnel: w507 -> [w508 w512]
            tunnel: [w508 w511] -> w506
            tunnel: w505 -> [_ w510]
            tunnel: [_ w509] -> w503
            frame False {
            }
            frame True {
              n179 = call "IPS magnet power supply - send GPIB cmd.vi"("error in (no error)"=w512, "Cmd string"=w510) -> ("error out"=w511:errorcluster, "Response"=w509:string)  [unwired: 8 in]
            }
          }
        }
      }
      n180 = call "Log commands.vi"("Log destination"=w488, "error in"=w487, "text to log"=w489) -> ("error out"=w486:errorcluster)  [unwired: 8 in]
    }
    frame "ToZeroField" {
      # "IPS\nNo arg"
      # "Check # of args"
      n181 = Equal?(x=0 ("y"), y=w524) -> (x = y?=w513:bool)
      n182 = case shown="True" w513 {
        tunnel: [w526 w532] -> w517
        tunnel: w522 -> [w528 w534]
        tunnel: [w528 w533] -> w515
        tunnel: w521 -> [w527 w532]
        tunnel: w520 -> [_ w531]
        tunnel: w519 -> [w525 _]
        tunnel: w518 -> [_ _]
        frame False {
          n183 = Merge Errors(w528, w525) -> ()  [unwired: 1 out]
          n184 = Unbundle By Name(w525) -> ("source"=w529:string)
          n185 = Concatenate Strings(w529, " : " ("string"), w527) -> (w526:string)
        }
        frame True {
          n186 = case shown="True" w531 {
            tunnel: w534 -> [w535 w538]
            tunnel: [w535 w537] -> w533
            tunnel: w532 -> [_ w536]
            frame False {
            }
            frame True {
              n187 = call "IPS magnet power supply - send GPIB cmd.vi"("error in (no error)"=w538, "Cmd string"=w536) -> ("error out"=w537:errorcluster)  [unwired: 8 in, 1 out]
            }
          }
        }
      }
      n188 = call "Log commands.vi"("Log destination"=w516, "error in"=w515, "text to log"=w517) -> ("error out"=w514:errorcluster)  [unwired: 8 in]
    }
    frame "HoldField" {
      # "IPS\nNo arg"
      # "Check # of args"
      n189 = Equal?(x=0 ("y"), y=w550) -> (x = y?=w539:bool)
      n190 = case shown="True" w539 {
        tunnel: [w552 w558] -> w543
        tunnel: w548 -> [w554 w560]
        tunnel: [w554 w559] -> w541
        tunnel: w547 -> [w553 w558]
        tunnel: w546 -> [_ w557]
        tunnel: w545 -> [w551 _]
        tunnel: w544 -> [_ _]
        frame False {
          n191 = Merge Errors(w554, w551) -> ()  [unwired: 1 out]
          n192 = Unbundle By Name(w551) -> ("source"=w555:string)
          n193 = Concatenate Strings(w555, " : " ("string"), w553) -> (w552:string)
        }
        frame True {
          n194 = case shown="True" w557 {
            tunnel: w560 -> [w561 w564]
            tunnel: [w561 w563] -> w559
            tunnel: w558 -> [_ w562]
            frame False {
            }
            frame True {
              n195 = call "IPS magnet power supply - send GPIB cmd.vi"("error in (no error)"=w564, "Cmd string"=w562) -> ("error out"=w563:errorcluster)  [unwired: 8 in, 1 out]
            }
          }
        }
      }
      n196 = call "Log commands.vi"("Log destination"=w542, "error in"=w541, "text to log"=w543) -> ("error out"=w540:errorcluster)  [unwired: 8 in]
    }
    frame "FieldScan" {
      # "Check # of args"
      # "IPS\nArg 1 : start field Bs [T]\nArg 2 : end field Be [T]\nArg 3 : sweep rate ->Bs [T/min]\nArg 4 : sweep rate Bs->Be [T/min]"
      n197 = Index Array(array=w596, index #1=0 ("index")) -> (element #1=w593:string, element #2=w589:string, element #3=w578:string, element #4=w577:string)  [unwired: 3 in]
      n198 = call "Check string represents a number.vi"("String"=w593) -> ("Is a number"=w575:bool, "Number"=w592:dbl)  [unwired: 13 in]
      n199 = call "Check string represents a number.vi"("String"=w578) -> ("Is a number"=w573:bool, "Number"=w584:dbl)  [unwired: 13 in]
      n200 = call "Check string represents a number.vi"("String"=w577) -> ("Is a number"=w572:bool, "Number"=w579:dbl)  [unwired: 13 in]
      n201 = call "Check string represents a number.vi"("String"=w589) -> ("Is a number"=w574:bool, "Number"=w586:dbl)  [unwired: 13 in]
      n202 = Equal?(x=4 ("y"), y=w585) -> (x = y?=w576:bool)
      n203 = In Range and Coerce(upper limit=18.0 ("lower limit"), x=w592, lower limit=0.0) -> (In Range?=w571:bool)  [unwired: 1 out]
      n204 = In Range and Coerce(upper limit=0.05 ("lower limit"), x=w584, lower limit=0.0) -> (In Range?=w569:bool)  [unwired: 1 out]
      n205 = In Range and Coerce(upper limit=0.05 ("lower limit"), x=w579, lower limit=0.0) -> (In Range?=w568:bool)  [unwired: 1 out]
      n206 = In Range and Coerce(upper limit=18.0 ("lower limit"), x=w586, lower limit=0.0) -> (In Range?=w570:bool)  [unwired: 1 out]
      n207 = Compound Arithmetic op=AND(w576, w575, w574, w573, w572) -> (w566:bool)
      n208 = Compound Arithmetic op=AND(w571, w570, w569, w568) -> (w567:bool)
      n209 = Compound Arithmetic op=AND(w566, w567) -> (w602:bool)
      n210 = case shown="True" w602 {
        tunnel: w598 -> [w612 w620]
        tunnel: [w604 w621] -> w597
        tunnel: w595 -> [w611 w617]
        tunnel: w594 -> [_ w619]
        tunnel: w591 -> [w616 _]
        tunnel: w590 -> [w615 _]
        tunnel: w566 -> [w608 _]
        tunnel: w565 -> [w606 w618]
        frame False {
          n211 = Not(x=w608) -> (.not. x?=w609:bool)
          n212 = Select(t=w616, s=w609, f=w615) -> (s? t:f=w610:errorcluster)
          n213 = Merge Errors(w612, w610) -> (w605:errorcluster)
          n214 = Unbundle By Name(w610) -> ("source"=w613:string)
          n215 = Concatenate Strings(w613, " : " ("string"), w611) -> (w607:string)
          n216 = call "Log commands.vi"("Log destination"=w606, "error in"=w605, "text to log"=w607) -> ("error out"=w604:errorcluster)  [unwired: 8 in]
        }
        frame True {
          n217 = case shown="True" w619 {
            tunnel: [w622 w624] -> w621
            tunnel: w620 -> [w622 w625]
            tunnel: w617 -> [_ w623]
            frame False {
            }
            frame True {
              # "Rem: this sub-vi will add\nother text to the log"
              n218 = call "Fieldscan measurement.vi"("error in (no error)"=w625, "Cmd string"=w623) -> ("error out"=w624:errorcluster)  [unwired: 8 in, 1 out]
            }
          }
          n219 = call "Log commands.vi"("Log destination"=w618, "text to log"=w617) -> ()  [unwired: 9 in, 1 out]
        }
      }
    }
    frame "--- Lakeshore ---" {
      # "separator"
    }
    frame "SetChannelA" {
      # "Check # of args"
      # "Lakeshore A\nArg 1 : channel number"
      n220 = Index Array(array=w647, index=0) -> (element=w639:string)
      n221 = call "Check string represents a number.vi"("String"=w639) -> ("Is a number"=w630:bool, "Number"=w638:dbl)  [unwired: 13 in]
      n222 = Equal?(x=1 ("y"), y=w646) -> (x = y?=w631:bool)
      n223 = Compound Arithmetic op=AND(w631, w630) -> (w627:bool)
      n224 = In Range and Coerce(upper limit=16 ("lower limit"), x=w638, lower limit=1) -> (In Range?=w629:bool)  [unwired: 1 out]
      n225 = Compound Arithmetic op=AND(w627, w629) -> (w628:bool)
      n226 = case shown="False" w628 {
        tunnel: [w651 w661] -> w635
        tunnel: w638 -> [_ w660]
        tunnel: w642 -> [w653 w663]
        tunnel: [w653 w662] -> w633
        tunnel: w641 -> [w652 w661]
        tunnel: w640 -> [_ w659]
        tunnel: w637 -> [w658 _]
        tunnel: w636 -> [w657 _]
        tunnel: w627 -> [w650 _]
        frame False {
          n227 = Not(x=w650) -> (.not. x?=w649:bool)
          n228 = Select(t=w658, s=w649, f=w657) -> (s? t:f=w654:errorcluster)
          n229 = Merge Errors(w653, w654) -> ()  [unwired: 1 out]
          n230 = Unbundle By Name(w654) -> ("source"=w655:string)
          n231 = Concatenate Strings(w655, " : " ("string"), w652) -> (w651:string)
        }
        frame True {
          n232 = case shown="True" w659 {
            tunnel: w663 -> [w664 w665]
            tunnel: [w664 w665] -> w662
            tunnel: w660 -> [_ w666]
            frame False {
            }
            frame True {
              n233 = global write "_Global variables 1.vi" "Lakeshore A channel"(w666) -> ()
            }
          }
        }
      }
      n234 = call "Log commands.vi"("Log destination"=w634, "error in"=w633, "text to log"=w635) -> ("error out"=w632:errorcluster)  [unwired: 8 in]
    }
    frame "SetChannelB" {
      # "Check # of args"
      # "Lakeshore B\nArg 1 : channel number"
      n235 = Index Array(array=w687, index=0) -> (element=w679:string)
      n236 = call "Check string represents a number.vi"("String"=w679) -> ("Is a number"=w670:bool, "Number"=w678:dbl)  [unwired: 13 in]
      n237 = Equal?(x=1 ("y"), y=w686) -> (x = y?=w671:bool)
      n238 = Compound Arithmetic op=AND(w671, w670) -> (w667:bool)
      n239 = In Range and Coerce(upper limit=16 ("lower limit"), x=w678, lower limit=1) -> (In Range?=w669:bool)  [unwired: 1 out]
      n240 = Compound Arithmetic op=AND(w667, w669) -> (w668:bool)
      n241 = case shown="True" w668 {
        tunnel: [w691 w701] -> w675
        tunnel: w678 -> [_ w700]
        tunnel: w682 -> [w693 w703]
        tunnel: [w693 w702] -> w673
        tunnel: w681 -> [w692 w701]
        tunnel: w680 -> [_ w699]
        tunnel: w677 -> [w698 _]
        tunnel: w676 -> [w697 _]
        tunnel: w667 -> [w690 _]
        frame False {
          n242 = Not(x=w690) -> (.not. x?=w689:bool)
          n243 = Select(t=w698, s=w689, f=w697) -> (s? t:f=w694:errorcluster)
          n244 = Merge Errors(w693, w694) -> ()  [unwired: 1 out]
          n245 = Unbundle By Name(w694) -> ("source"=w695:string)
          n246 = Concatenate Strings(w695, " : " ("string"), w692) -> (w691:string)
        }
        frame True {
          n247 = case shown="True" w699 {
            tunnel: w703 -> [w704 w705]
            tunnel: [w704 w705] -> w702
            tunnel: w700 -> [_ w706]
            frame False {
            }
            frame True {
              n248 = global write "_Global variables 1.vi" "Lakeshore B channel"(w706) -> ()
            }
          }
        }
      }
      n249 = call "Log commands.vi"("Log destination"=w674, "error in"=w673, "text to log"=w675) -> ("error out"=w672:errorcluster)  [unwired: 8 in]
    }
    frame "GetTempA" {
      # "Lakeshore A\nInput : no argument"
      n250 = case shown="True" w707 {
        tunnel: w710 -> [w711 w716]
        tunnel: [w711 w715] -> w709
        tunnel: [_ w712] -> w708
        frame False {
        }
        frame True {
          n251 = call "Lakeshore 370 - send GPIB cmd.vi"("Lakeshore device"=Lakeshore_device_selector."A", "error in (no error)"=w716, "Cmd string"="GetTemp") -> ("error out"=w715:errorcluster, "Response"=w712:string)  [unwired: 7 in]
        }
      }
    }
    frame "GetTempB" {
      # "Lakeshore B\nInput : no argument"
      n252 = case shown="True" w717 {
        tunnel: w720 -> [w721 w726]
        tunnel: [w721 w725] -> w719
        tunnel: [_ w722] -> w718
        frame False {
        }
        frame True {
          n253 = call "Lakeshore 370 - send GPIB cmd.vi"("Lakeshore device"=Lakeshore_device_selector."B", "error in (no error)"=w726, "Cmd string"="GetTemp") -> ("error out"=w725:errorcluster, "Response"=w722:string)  [unwired: 7 in]
        }
      }
    }
    frame "--- Device X ---" {
      # "separator"
    }
    frame "--- Device Y ---" {
      # "separator"
    }
    frame "--- Device Z ---" {
      # "separator"
    }
  }
  "error out" <- w13
  "Response" <- w12
